vi "Filter Get Threshold.vi"(11 "threshold":sgl) -> (2 "function return":u32, 3 "threshold out":sgl)   [LabVIEW 2018, in "Copy of Andor SDK.lvlib"]
doc: "EXPNETTYPE unsigned int WINAPI Filter_GetThreshold(float * threshold);"
uses:
  Copy of Andor SDK.lvlib
  <userlib>/Andor SDK/ATMCD32D.dll
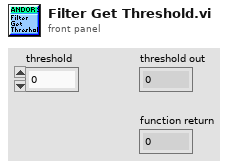
[diagram p1: front panel]
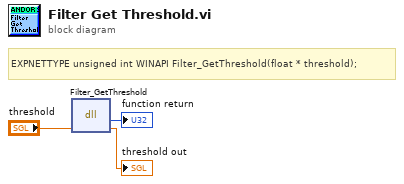
[diagram p0: block diagram]
diagram:
  # "EXPNETTYPE unsigned int WINAPI Filter_GetThreshold(float * threshold);"
  n1 = dll-call lib="C:/Program Files (x86)/National Instruments/LabVIEW 2018/user.lib/Andor SDK/ATMCD32D.*" fn="Filter_GetThreshold"("threshold"="threshold") -> (→"function return":u32, "threshold"=→"threshold out":sgl)  [unwired: 3 in, 2 out]
